vi "_079.vi"() -> ()   [LabVIEW 2024]
panel:
  out "output array":i32[][](array[numeric])
  out "output array":i32[][](array[numeric])
  # "Fundamentals :"
  # "8~>After running this VI,what is the value displayed in the o/p ?"
  # "Nrml Approach :"
  # "Dfrnt Approach :"
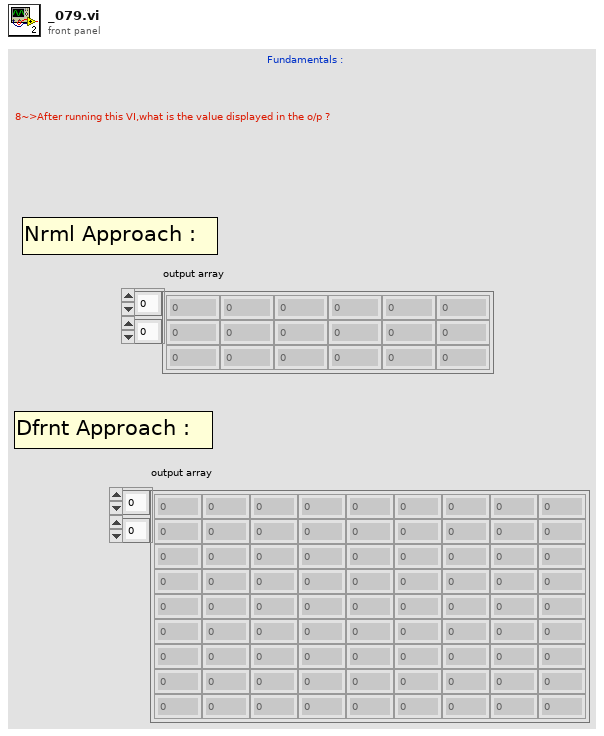
[diagram p1: front panel]
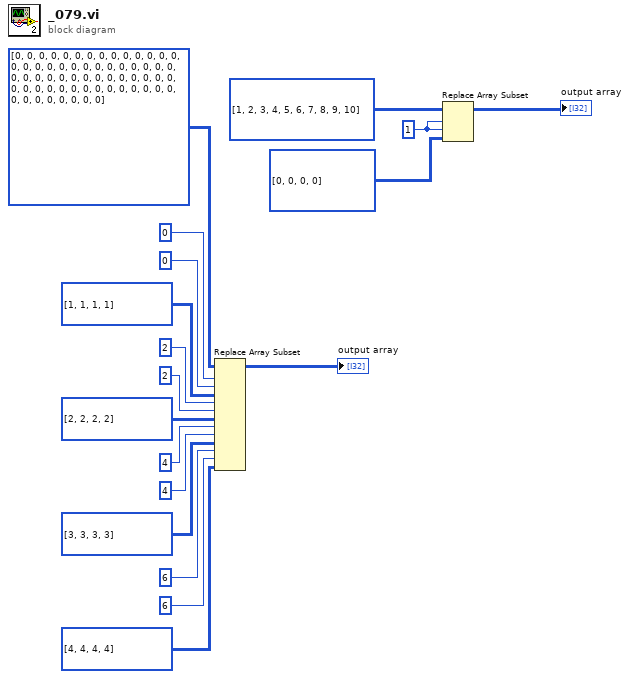
[diagram p0: block diagram]
diagram:
  w11 = 1
  n1 = Replace Array Subset "Replace Array Subset"(array=i32[][] [[0, 0, 0, 0, 0, 0, 0, 0], [0, 0, 0, 0, 0, 0, 0, 0], [0, 0, 0, 0, 0, 0, 0, 0], [0, 0, 0, 0, 0, 0, 0, 0], [0, 0, 0, 0, 0, 0, 0, 0], [0, 0, 0, 0, 0, 0, 0, 0], [0, 0, 0, 0, 0, 0, 0, 0], [0, 0, 0, 0, 0, 0, 0, 0]], new element #1=i32[][] [[1, 1], [1, 1]], index (row) #1=0, index (col) #1=0, new element #2=i32[][] [[2, 2], [2, 2]], index (row) #2=2, index (col) #2=2, new element #3=i32[][] [[3, 3], [3, 3]], index (row) #3=4, index (col) #3=4, new element #4=i32[][] [[4, 4], [4, 4]], index (row) #4=6, index (col) #4=6) -> (→"output array":i32[][])
  n2 = Replace Array Subset "Replace Array Subset"(array=i32[][] [[1, 2, 3, 4, 5], [6, 7, 8, 9, 10]], new element=i32[][] [[0, 0], [0, 0]], index (row)=w11, index (col)=w11) -> (→"output array":i32[][])
